vi "Transform Components to Transformation Matrix.vi"(1 "Rotation Matrix in":T1, 2 "tvec":T2) -> (0 "4x4 Transformation Matrix":T1)   [LabVIEW 2020, in "ar.lvlib"]
doc: "Convert tvec and a rotation matrix to a 4x4 transformation matrix."
uses:
  ar.lvlib
  <vilib>/Analysis/Matrix/Datatypes/RealMatrix.ctl
  <vilib>/Analysis/Matrix/NI_Matrix.lvlib
  tvec.ctl
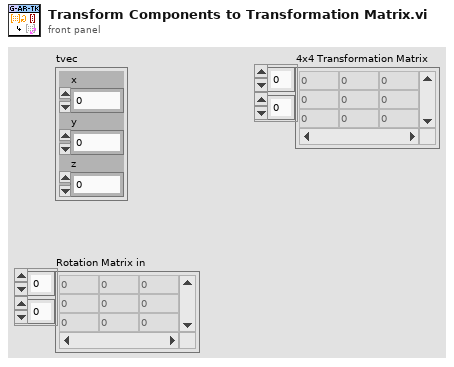
[diagram p1: front panel]
types:
  T1 = typedef "NI_Matrix.lvlib/RealMatrix.ctl" = dbl[][]
  T2 = typedef "ar.lvlib/tvec.ctl" = cluster{"x":dbl, "y":dbl, "z":dbl}
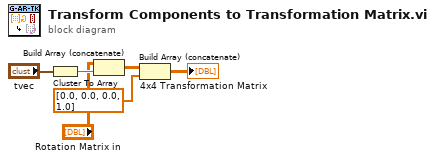
[diagram p0: block diagram]
diagram:
  n1 = Cluster To Array(cluster="tvec") -> (array=w2:dbl[])
  n2 = Build Array (concatenate)("Rotation Matrix in", w2) -> (w4:T1)
  n3 = Build Array (concatenate)(w4, dbl[] [0.0, 0.0, 0.0, 1.0]) -> (→"4x4 Transformation Matrix":T1)
